vi "LJstreamM tc formula handler.vi"(5 "Input Values In":dbl[][](array[numeric]) format="%.2f", 6 "error in (no error)":errorcluster, 7 "formula":string, 8 "Variables Input":string[](array[string])=["v1", "v2", "v3", "v4"], 9 "Index":i32) -> (0 "error out":errorcluster, 1 "formula out":string, 4 "Input Values Out":dbl[][](array[numeric]) format="%.2f")   [LabVIEW 2025]
doc: "Similar to the Formula Node function, but with variables that can be entered on the front panel."
panel:
  out "Computed Values":dbl[][](array[numeric])
  out "Executed\nFunction":string
  # "Input = v\nOutput = y"
  # "y=TCVoltsToTemp[J:z:z];"
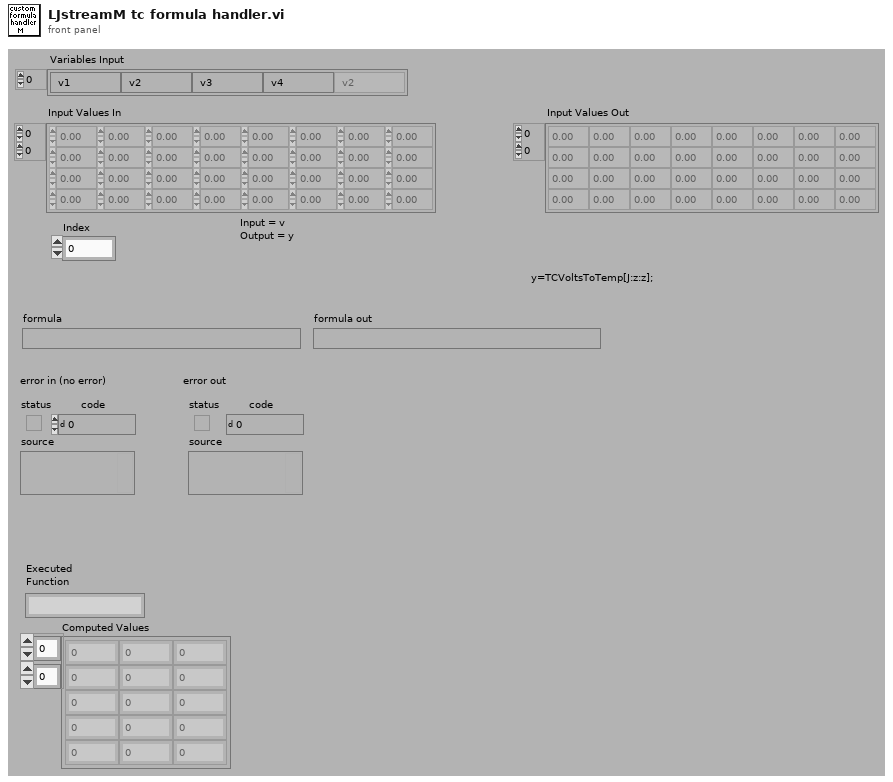
[diagram p1: front panel]
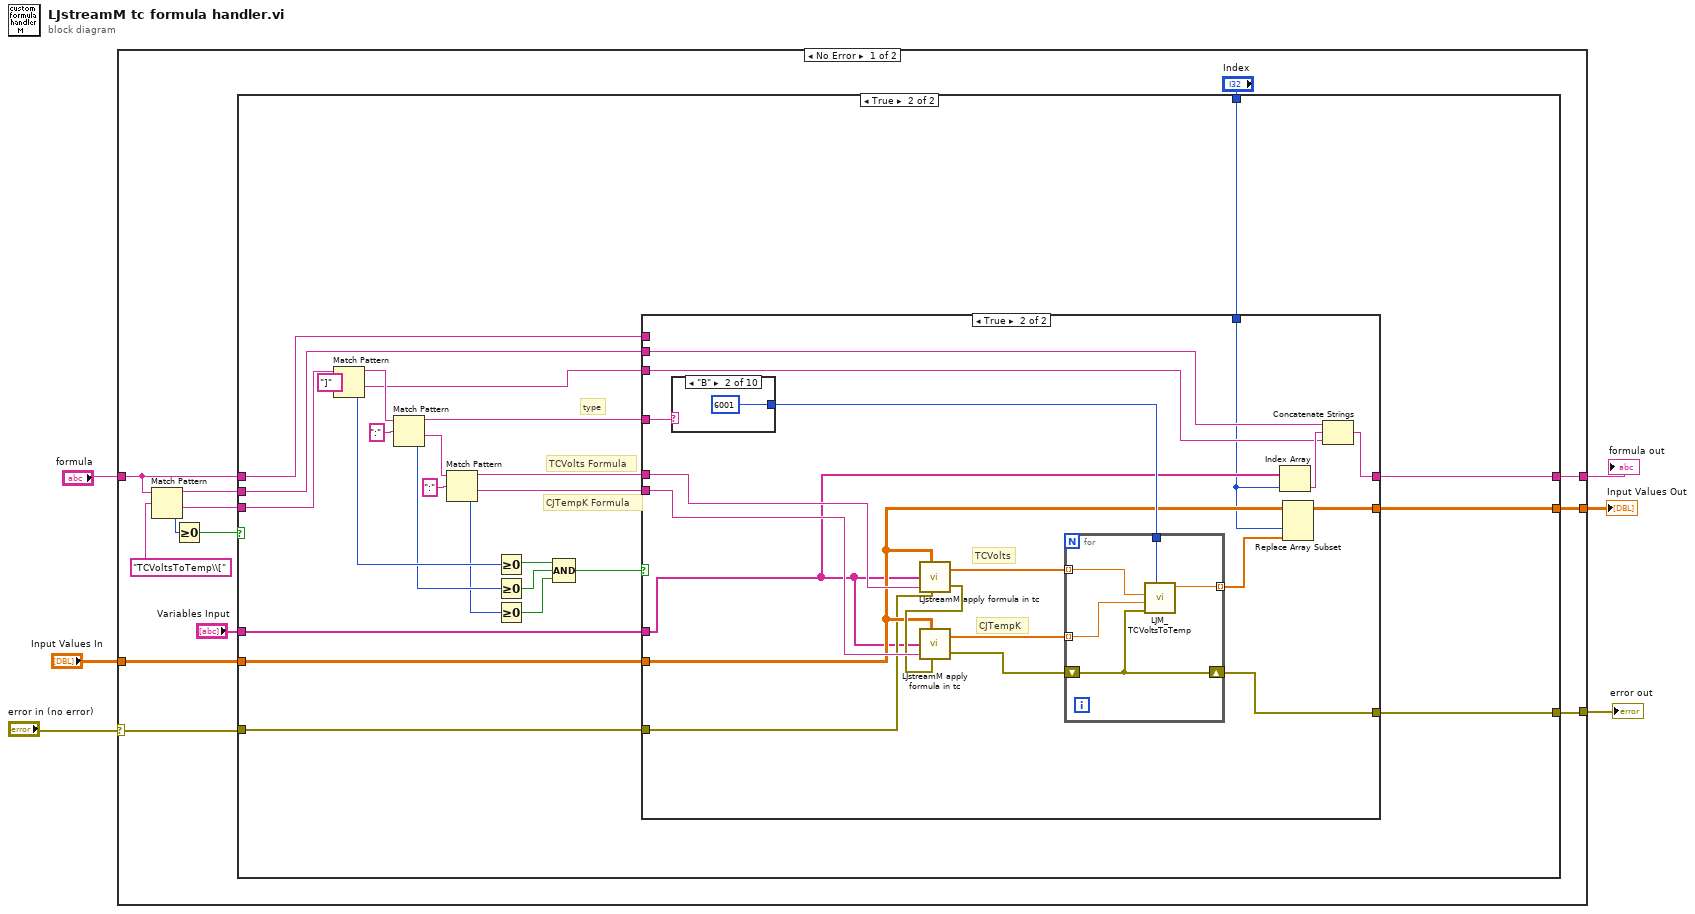
[diagram p0: block diagram]
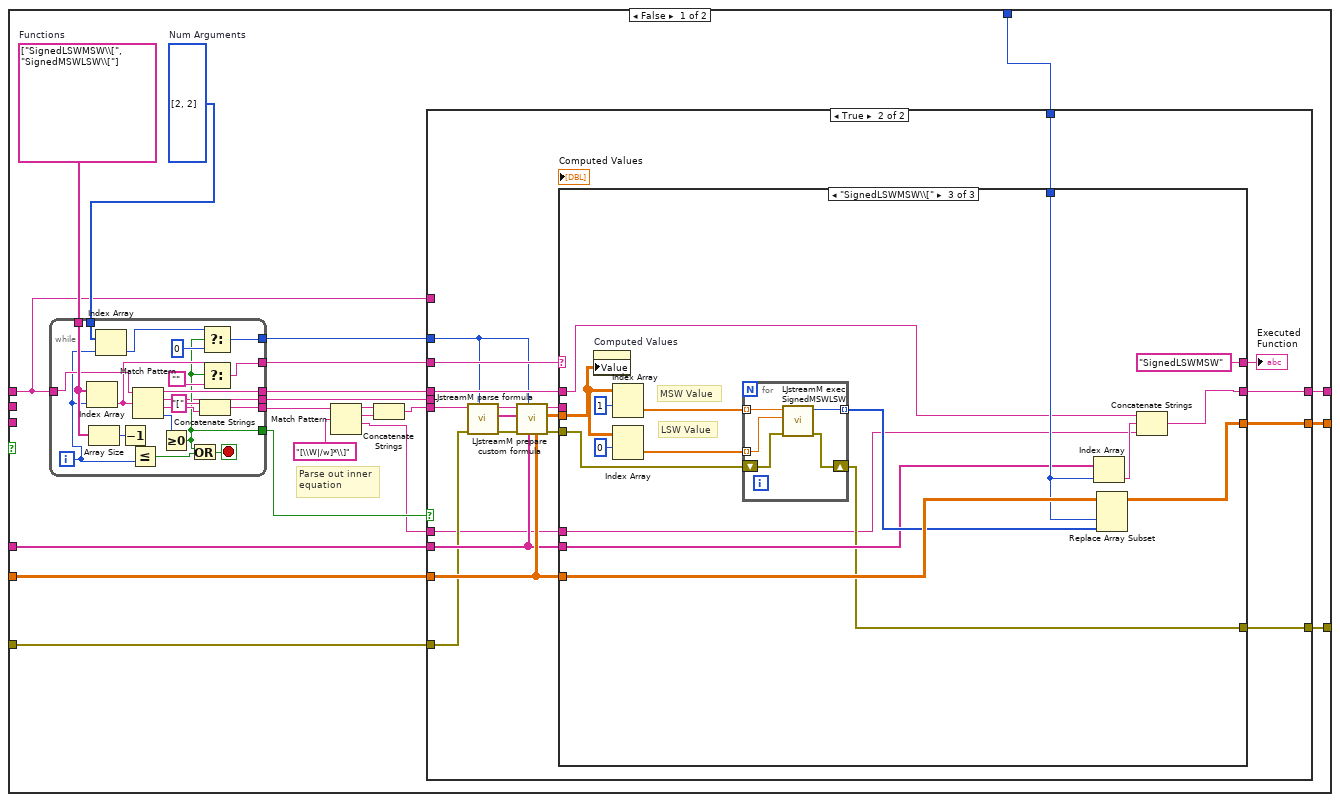
[diagram p2: hidden frame]
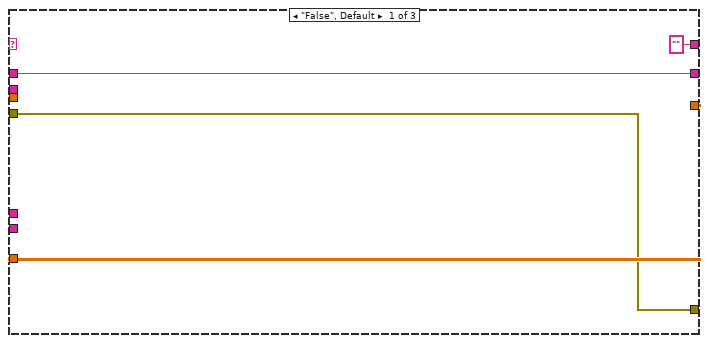
[diagram p4: hidden frame]
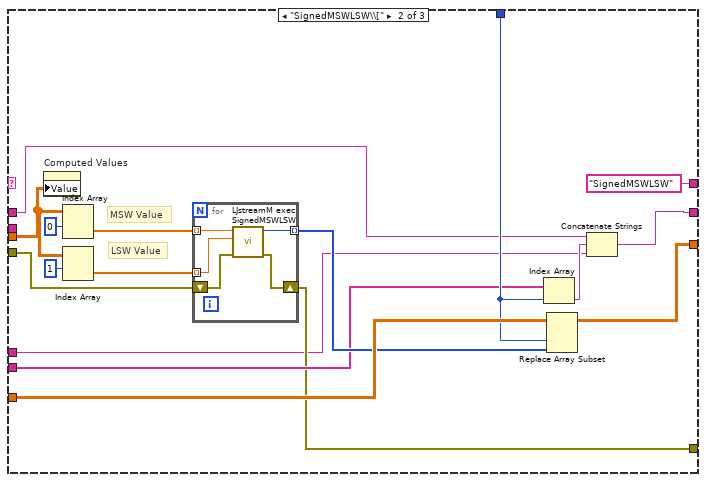
[diagram p5: hidden frame]
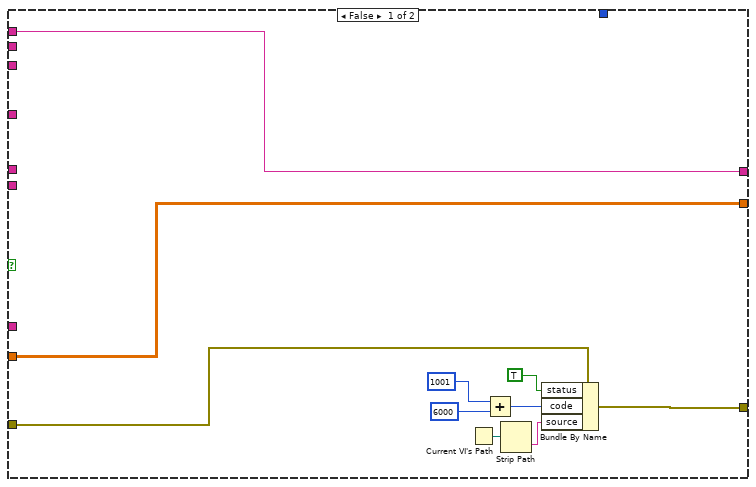
[diagram p6: hidden frame]
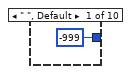
[diagram p7: hidden frame]
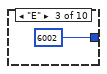
[diagram p8: hidden frame]
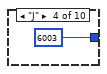
[diagram p9: hidden frame]
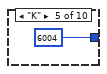
[diagram p10: hidden frame]
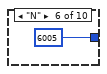
[diagram p11: hidden frame]
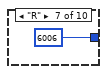
[diagram p12: hidden frame]
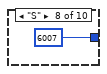
[diagram p13: hidden frame]
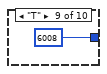
[diagram p14: hidden frame]
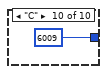
[diagram p15: hidden frame]
diagram:
  n1 = case shown="No Error" "error in (no error)" {
    selector: "error in (no error)" -> [w10 w202]
    tunnel: "formula" -> [w16 w204]
    tunnel: "Input Values In" -> [w13 w203]
    tunnel: [w12 w203] -> w4
    tunnel: [w11 w204] -> w3
    tunnel: [w9 w202] -> w1
    frame No Error {
      n2 = Match Pattern(string=w16, regular expression="TCVoltsToTemp\\[") -> (before substring=w15:string, after substring=w14:string, offset past match=w17:i32)  [unwired: 1 in, 1 out]
      n3 = Greater Or Equal To 0?(x=w17) -> (x >= 0?=w18:bool)
      n4 = case shown="True" w18 {
        tunnel: w16 -> [w27 w136]
        tunnel: [w39 w137] -> w11
        tunnel: w15 -> [_ w138]
        tunnel: w14 -> [_ w157]
        tunnel: w13 -> [w33 w141]
        tunnel: [w40 w140] -> w12
        tunnel: w10 -> [w30 w135]
        tunnel: [w29 w134] -> w9
        tunnel: "Variables Input" -> [w31 w133]
        tunnel: "Index" -> [w32 w132]
        frame False {
          w35 = i32[] [2, 2]  # Num Arguments
          w38 = string[] ["SignedLSWMSW\\[", "SignedMSWLSW\\["]  # Functions
          # "Parse out inner\nequation"
          n5 = while {
            tunnel: w38 -> [w130]
            tunnel: [w127] -> w36
            tunnel: w27 -> [w126]
            tunnel: [w122] -> w37
            tunnel: [w115] -> w25
            tunnel: w35 -> [w120]
            tunnel: [w116] -> w34
            tunnel: [w112] -> w28
            tunnel: [w111] -> w26
            i -> [w119]
            stop <- w129 stop-if-true
            n6 = Index Array(array=w130, index=w119) -> (element=w123:string)
            n7 = Array Size(array=w130) -> (size(s)=w125:i32)
            n8 = Index Array(array=w120, index=w119) -> (element=w117:i32)
            n9 = Decrement(x=w125) -> (x-1=w124:i32)
            n10 = Less Or Equal?(x=w124, y=w119) -> (x <= y?=w131:bool)
            n11 = Match Pattern(string=w126, regular expression=w123) -> (before substring=w127:string, match substring=w111:string, after substring=w113:string, offset past match=w128:i32)  [unwired: 1 in]
            n12 = Greater Or Equal To 0?(x=w128) -> (x >= 0?=w112:bool)
            n13 = Or(x=w112, y=w131) -> (x .or. y?=w129:bool)
            n14 = Concatenate Strings("[" ("string"), w113) -> (w115:string)
            n15 = Select(t=w117, s=w112, f=0) -> (s? t:f=w116:i32)
            n16 = Select(t=w123, s=w112, f="") -> (s? t:f=w122:string)
          }
          n17 = Match Pattern(string=w25, regular expression="[\\W|/w]*\\]") -> (before substring=w23:string, match substring=w21:string, after substring=w20:string)  [unwired: 1 in, 1 out]
          n18 = Concatenate Strings(w23, w21) -> (w22:string)
          n19 = case shown="True" w28 {
            tunnel: [w42 w62] -> w40
            tunnel: [w41 w61] -> w39
            tunnel: w37 -> [_ w60]
            tunnel: w36 -> [_ w58]
            tunnel: w22 -> [_ w45]
            tunnel: w34 -> [_ w54]
            tunnel: w33 -> [w42 w50]
            tunnel: w32 -> [_ w49]
            tunnel: w31 -> [_ w48]
            tunnel: w30 -> [w43 w47]
            tunnel: [w43 w46] -> w29
            tunnel: w27 -> [w41 _]
            tunnel: w26 -> [_ _]
            tunnel: w20 -> [_ w44]
            frame False {
            }
            frame True {
              n20 = call "LJstreamM parse formula.vi"("Num Args"=w54, "error in (no error)"=w47, "Input Formula"=w45) -> ("error out"=w55:errorcluster, "Output Formula Arguments"=w56:string[], "Output Formula"=w57:string)  [unwired: 6 in]
              n21 = call "LJstreamM prepare custom formula.vi"("Input Values"=w50, "Variables Input"=w48, "NumFormulas"=w54, "error in (no error)"=w55, "formulas"=w56, "Input Formula"=w57) -> ("error out"=w51:errorcluster, "Computed Values"=w52:dbl[][], "Output Formula"=w53:string)  [unwired: 3 in]
              n22 = case shown="\"SignedLSWMSW\\\\[\"" w60 {
                tunnel: w58 -> [w65 w70 w92]
                tunnel: w50 -> [w66 w75 w97]
                tunnel: [w66 w74 w96] -> w62
                tunnel: [w65 w73 w95] -> w61
                tunnel: ["" "SignedMSWLSW" "SignedLSWMSW"] -> w59
                tunnel: w53 -> [_ _ _]
                tunnel: w52 -> [_ w80 w102]
                tunnel: w51 -> [w63 w77 w99]
                tunnel: w49 -> [_ w72 w94]
                tunnel: w48 -> [_ w69 w91]
                tunnel: [w63 w68 w90] -> w46
                tunnel: w44 -> [_ w67 w89]
                frame "False", Default {
                }
                frame "SignedMSWLSW\\[" {
                  # "LSW Value"
                  # "MSW Value"
                  n23 = property on="Computed Values" class="Arr (strict)"("Value"=w80) -> ()  [unwired: 2 in, 2 out]
                  n24 = Index Array(array=w80, index (row)=0) -> (element=w79:dbl[])  [unwired: 1 in]
                  n25 = Index Array(array=w80, index (row)=1) -> (element=w78:dbl[])  [unwired: 1 in]
                  n26 = for {
                    tunnel: w79 -> [w85] mode=indexing
                    tunnel: w78 -> [w84] mode=indexing
                    shift-right: [w87] -> w68
                    shift-left: w77 -> [w88]
                    tunnel: [w86] -> w71 mode=indexing
                    n27 = call "LJstreamM exec SignedMSWLSW.vi"("error in (no error)"=w88, "LSB"=w84, "MSB"=w85) -> ("error out"=w87:errorcluster, "(MSB << 16 ) | LSB"=w86:u32)  [unwired: 7 in]
                  }
                  n28 = Index Array(array=w69, index=w72) -> (element=w76:string)
                  n29 = Replace Array Subset(array=w75, new element=w71, index (col)=w72) -> (w74:dbl[][])  [unwired: 1 in]
                  n30 = Concatenate Strings(w70, w76, w67) -> (w73:string)
                }
                frame "SignedLSWMSW\\[" {
                  # "LSW Value"
                  # "MSW Value"
                  n31 = property on="Computed Values" class="Arr (strict)"("Value"=w102) -> ()  [unwired: 2 in, 2 out]
                  n32 = Index Array(array=w102, index (row)=1) -> (element=w101:dbl[])  [unwired: 1 in]
                  n33 = Index Array(array=w102, index (row)=0) -> (element=w100:dbl[])  [unwired: 1 in]
                  n34 = for {
                    tunnel: w101 -> [w107] mode=indexing
                    tunnel: w100 -> [w106] mode=indexing
                    shift-right: [w109] -> w90
                    shift-left: w99 -> [w110]
                    tunnel: [w108] -> w93 mode=indexing
                    n35 = call "LJstreamM exec SignedMSWLSW.vi"("error in (no error)"=w110, "LSB"=w106, "MSB"=w107) -> ("error out"=w109:errorcluster, "(MSB << 16 ) | LSB"=w108:u32)  [unwired: 7 in]
                  }
                  n36 = Index Array(array=w91, index=w94) -> (element=w98:string)
                  n37 = Replace Array Subset(array=w97, new element=w93, index (col)=w94) -> (w96:dbl[][])  [unwired: 1 in]
                  n38 = Concatenate Strings(w92, w98, w89) -> (w95:string)
                }
              }
              "Executed\nFunction" <- w59
            }
          }
        }
        frame True {
          # "CJTempK Formula"
          # "TCVolts Formula"
          # "type"
          n39 = Match Pattern(string=w157, regular expression="]") -> (before substring=w155:string, after substring=w139:string, offset past match=w151:i32)  [unwired: 1 in, 1 out]
          n40 = Match Pattern(string=w155, regular expression=":") -> (before substring=w144:string, after substring=w152:string, offset past match=w150:i32)  [unwired: 1 in, 1 out]
          n41 = Match Pattern(string=w152, regular expression=":") -> (before substring=w143:string, after substring=w142:string, offset past match=w149:i32)  [unwired: 1 in, 1 out]
          n42 = Greater Or Equal To 0?(x=w151) -> (x >= 0?=w148:bool)
          n43 = Greater Or Equal To 0?(x=w150) -> (x >= 0?=w147:bool)
          n44 = Greater Or Equal To 0?(x=w149) -> (x >= 0?=w146:bool)
          n45 = Compound Arithmetic op=AND(w148, w147, w146) -> (w145:bool)
          n46 = case shown="True" w145 {
            tunnel: w144 -> [_ w186]
            tunnel: w143 -> [_ w184]
            tunnel: w142 -> [_ w185]
            tunnel: w141 -> [w166 w178]
            tunnel: [w166 w176] -> w140
            tunnel: w139 -> [_ w174]
            tunnel: w138 -> [_ w173]
            tunnel: [w167 w168] -> w137
            tunnel: w136 -> [w167 _]
            tunnel: w135 -> [w161 w172]
            tunnel: [w160 w171] -> w134
            tunnel: w133 -> [_ w170]
            tunnel: w132 -> [_ w169]
            frame False {
              n47 = Current VI's Path() -> (path=w164:path)
              n48 = Add(x=1001, y=6000) -> (x+y=w163:i32)
              n49 = Strip Path(path=w164) -> (name=w165:string)  [unwired: 1 out]
              n50 = Bundle By Name(cluster=w161, "status"=TRUE, "code"=w163, "source"=w165) -> (w160:errorcluster)
            }
            frame True {
              # "CJTempK"
              # "TCVolts"
              n51 = case shown="\"B\"" w186 {
                tunnel: [-999 6001 6002 6003 6004 6005 6006 6007 6008 6009] -> w180
                frame " ", Default {
                }
                frame "B" {
                }
                frame "E" {
                }
                frame "J" {
                }
                frame "K" {
                }
                frame "N" {
                }
                frame "R" {
                }
                frame "S" {
                }
                frame "T" {
                }
                frame "C" {
                }
              }
              n52 = call "LJstreamM apply formula in tc.vi"("Input Values"=w178, "Variables Input"=w170, "formula"=w184, "error in (no error)"=w172) -> ("Output Values"=w182:dbl[], "error out"=w183:errorcluster)  [unwired: 1 in]
              n53 = call "LJstreamM apply formula in tc.vi"("Input Values"=w178, "Variables Input"=w170, "formula"=w185, "error in (no error)"=w183) -> ("Output Values"=w181:dbl[], "error out"=w179:errorcluster)  [unwired: 1 in]
              n54 = for {
                tunnel: w182 -> [w190] mode=indexing
                tunnel: w181 -> [w189] mode=indexing
                tunnel: w180 -> [w191]
                shift-right: [w187] -> w171
                shift-left: w179 -> [w187]
                tunnel: [w188] -> w177 mode=indexing
                n55 = call "LJM_TCVoltsToTemp.vi"("TCType"=w191, "error in"=w187, "CJTempK"=w189, "TCVolts"=w190) -> ("TCTempK"=w188:dbl)  [unwired: 4 in, 3 out]
              }
              n56 = Index Array(array=w170, index=w169) -> (element=w175:string)
              n57 = Replace Array Subset(array=w178, new element=w177, index (col)=w169) -> (w176:dbl[][])  [unwired: 1 in]
              n58 = Concatenate Strings(w173, w175, w174) -> (w168:string)
            }
          }
        }
      }
    }
    frame Error {
    }
  }
  "error out" <- w1
  "formula out" <- w3
  "Input Values Out" <- w4
